vi "Pre Launch Init.vi"(11 "Actor wHelper in":refnum<class "Actor wHelper.lvclass">) -> (0 "error out":errorcluster, 3 "Actor wHelper out":refnum<class "Actor wHelper.lvclass">)   [LabVIEW 2017, in "Framework.lvlib" / "Actor wHelper.lvclass"]
doc: "(<B>Filename</B>: Actor Framework.lvlib:Actor.lvclass:Pre Launch Init.vi)\n\nDefines behavior that occurs after the Launch Nested Actor method is invoked but before the actor's Actor Core method begins running.\n\nBy default, this method does nothing. A descendant class may override it to define behavior."
uses:
  Actor wHelper.lvclass
  Actor wHelper.lvclass/Actor wHelper.ctl
  Actor wLauncher/Actor wLauncher.lvclass
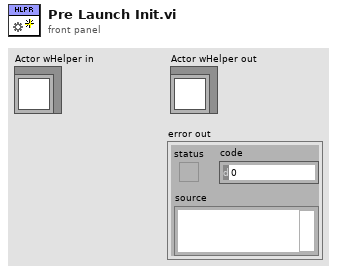
[diagram p1: front panel]
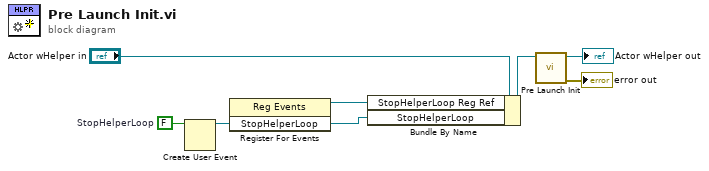
[diagram p0: block diagram]
diagram:
  w4 = FALSE  # StopHelperLoop
  n1 = Create User Event(user event datatype=w4) -> (user event=w2:refnum<user-event>)  [unwired: 1 in, 1 out]
  n2 = register-events(w2) -> (reference out=w1:refnum<event-registration>)  [unwired: 2 in, 1 out]
  n3 = Bundle By Name(cluster="Actor wHelper in", "StopHelperLoop Reg Ref"=w1, "StopHelperLoop"=w2) -> (w3:refnum<class "Actor wHelper.lvclass">)
  n4 = call-parent "Pre Launch Init.vi"("Actor wLauncher in"=w3) -> ("error out"=→"error out":errorcluster, "Actor wLauncher out"=→"Actor wHelper out":refnum<class "Actor wHelper.lvclass">)  [unwired: 9 in]
